vi "DPIDs.Compile.vi"(8 "error in (no error)":errorcluster, 10 "PIDs":T3[](array[typedef]) {"Signals"."Byte Order" items=["Little Endian", "Big Endian"]; "Signals"."Data Type" items=["Signed", "Unsigned", "IEEE Float"]}, 11 "DPIDs":T1[](array[typedef])) -> (0 "error out":errorcluster, 3 "Lookup Table":variant)   [LabVIEW 2019, in "Diagnostics Addon System Explorer.lvlib"]
uses:
  Shared/Types/Frame.Compile.ctl
  Shared/Types/Type.ctl
  Shared/Types/Signal.ctl
  Shared/Types/DPID.ctl
  Shared/Types/DPID.Rate.ctl
  Shared/Types/DPID.Lookup.Info.ctl
  Shared/Types/DPID.Lookup.Info.PID.ctl
  Diagnostics Addon System Explorer.lvlib
  Shared/Diagnostics Addon Shared.lvlib
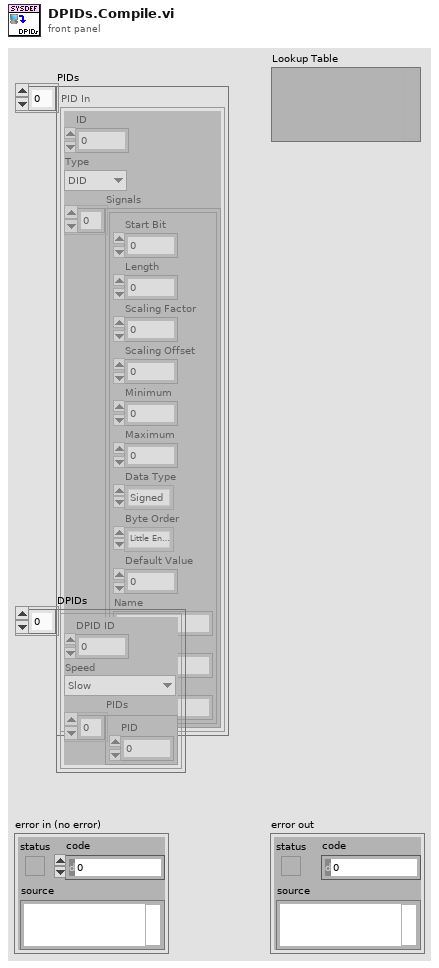
[diagram p1: front panel]
types:
  T1 = typedef "Diagnostics Addon Shared.lvlib/DPID.ctl" = cluster{"DPID ID":u8, "Speed":T2, "PIDs":u16[]}
  T2 = typedef "Diagnostics Addon Shared.lvlib/DPID.Rate.ctl" = enum16{"Slow", "Medium", "Fast"}
  T3 = typedef "Diagnostics Addon Shared.lvlib/Frame.Compile.ctl" = cluster{"ID":u32, "Type":T4, "Signals":T5[]}
  T4 = typedef "Diagnostics Addon Shared.lvlib/Type.ctl" = enum16{"DID", "CDID", "PID", "CPID", "Read Memory", "Write Memory", "IO Control", "Routine Start", "Routine Request", "Routine Stop", "User Defined", "DTC Control", "Clear DTCs", "Read DTCs", "Start DTCs", "DTC Change Count", "Tester Present", "Unlock ECU", "Reset ECU", "Diagnostic Session Control", "Normal Communication Control", "Configure and Start DPIDs", "Stop DPIDs"}
  T5 = typedef "Diagnostics Addon Shared.lvlib/Signal.ctl" = cluster{"Start Bit":u32, "Length":u32, "Scaling Factor":dbl, "Scaling Offset":dbl, "Minimum":dbl, "Maximum":dbl, "Data Type":u32, "Byte Order":u32, "Default Value":dbl, "Name":string, "Units":string, "Description":string}
  T6 = typedef "Diagnostics Addon Shared.lvlib/DPID.Lookup.Info.ctl" = cluster{"PID Info":T7}
  T7 = typedef "Diagnostics Addon Shared.lvlib/DPID.Lookup.Info.PID.ctl" = cluster{"PID":u16, "Frame Length":u8}
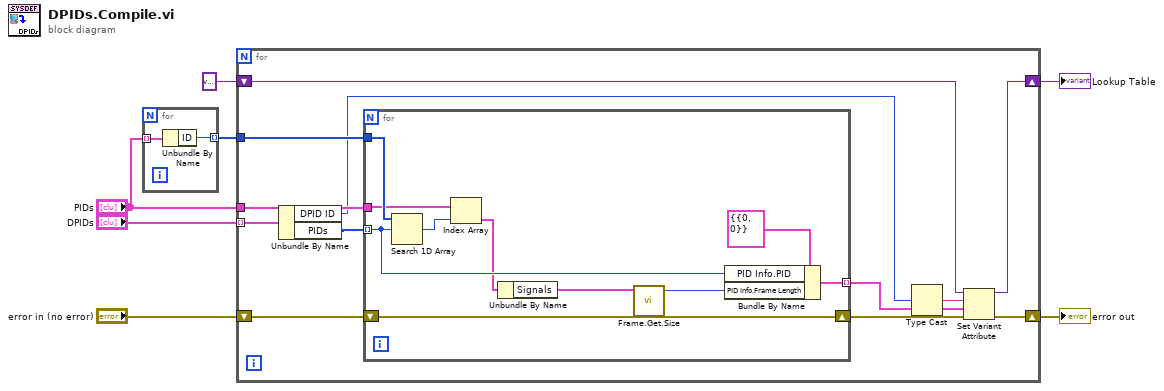
[diagram p0: block diagram]
diagram:
  n1 = for {
    tunnel: "PIDs" -> [w9] mode=indexing
    tunnel: [w8] -> w3 mode=indexing
    n2 = Unbundle By Name(w9) -> ("ID"=w8:u32)
  }
  n3 = for {
    tunnel: "DPIDs" -> [w21] mode=indexing
    tunnel: w3 -> [w20]
    tunnel: "PIDs" -> [w18]
    shift-right: [w11] -> w5
    shift-left: variant -> [w17]
    shift-right: [w12] -> w1
    shift-left: "error in (no error)" -> [w15]
    n4 = Unbundle By Name(w21) -> ("DPID ID"=w16:u8, "PIDs"=w19:u16[])
    n5 = for {
      tunnel: w20 -> [w31]
      tunnel: w19 -> [w27] mode=indexing
      tunnel: w18 -> [w30]
      shift-right: [w28] -> w14
      shift-left: w15 -> [w28]
      tunnel: [w26] -> w10 mode=indexing
      n6 = Search 1D Array(1D array=w31, element=w27) -> (index of element=w29:i32)  [unwired: 1 in]
      n7 = Index Array(array=w30, index=w29) -> (element=w24:T3)
      n8 = Unbundle By Name(w24) -> ("Signals"=w23:T5[])
      n9 = call "Frame.Get.Size.vi"("Parameters"=w23) -> ("Bytes"=w22:u32)  [unwired: 10 in]
      n10 = Bundle By Name(cluster=T6 {"PID Info"={"PID"=0, "Frame Length"=0}} ("Cluster"), "PID Info.PID"=w27, "PID Info.Frame Length"=w22) -> (w26:T6)
    }
    n11 = Type Cast(x=w16) -> (*(type *) &x=w13:string)  [unwired: 1 in]
    n12 = Set Variant Attribute(Variant=w17, name=w13, value=w10, error in=w14) -> (Variant out=w11:variant, error out=w12:errorcluster)  [unwired: 1 out]
  }
  "error out" <- w1
  "Lookup Table" <- w5
